vi "MainMesaurementDataPipe.vi"(8 "error in (no error)":errorcluster, 9 "WFChart Refnum":refnum<vi>, 10 "IntGraph Refnum in":refnum<vi>, 11 "IntensityGraph in":refnum<vi>) -> (0 "error out":errorcluster)   [LabVIEW 2013]
uses:
  Variables/GlobalCameraDebugTemperature.vi
  Variables/GlobalGetMesaurementStatus.vi
  Variables/GlobalSetGetPixelOfRoi.vi
  Variables/GlobalDevice.vi
  Variables/GlobalExitVar.vi
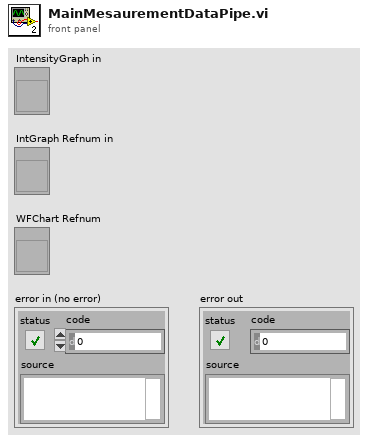
[diagram p1: front panel]
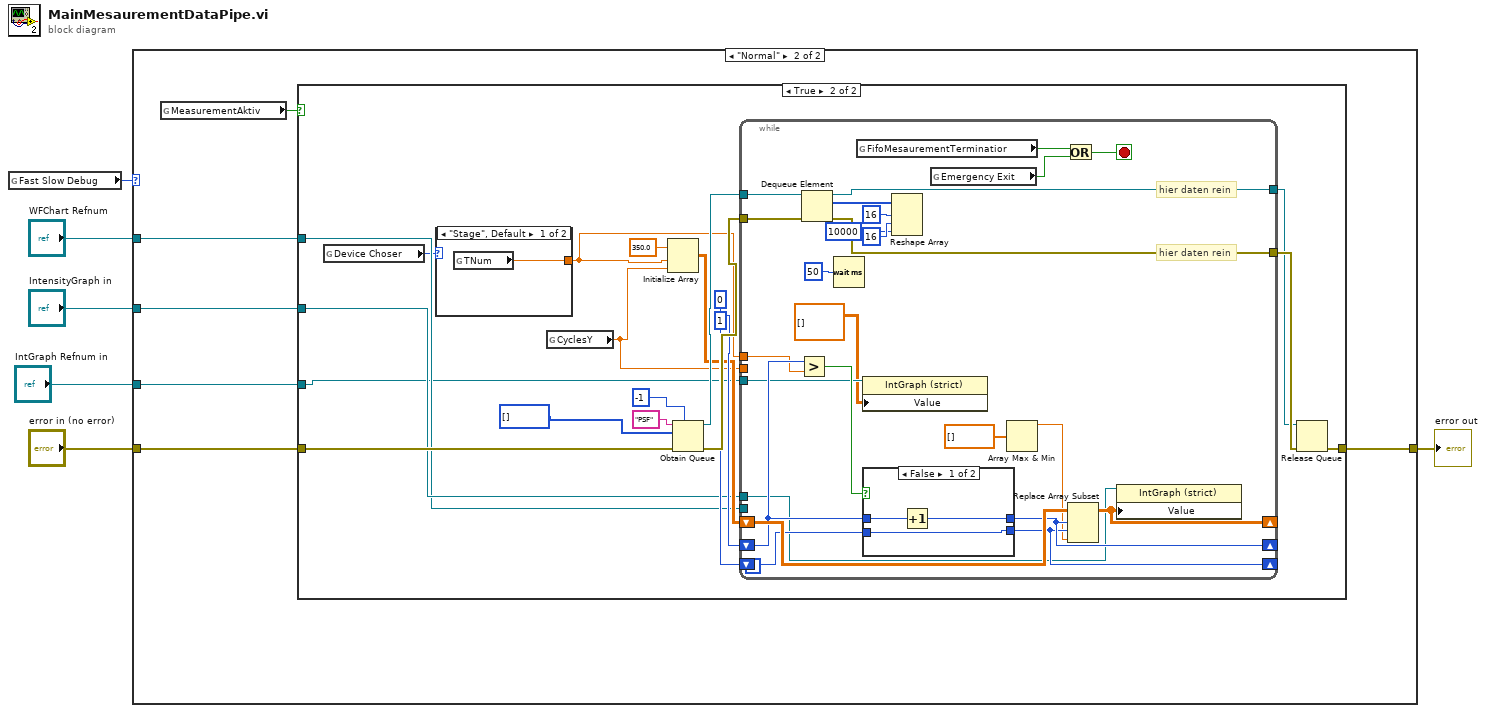
[diagram p0: block diagram]
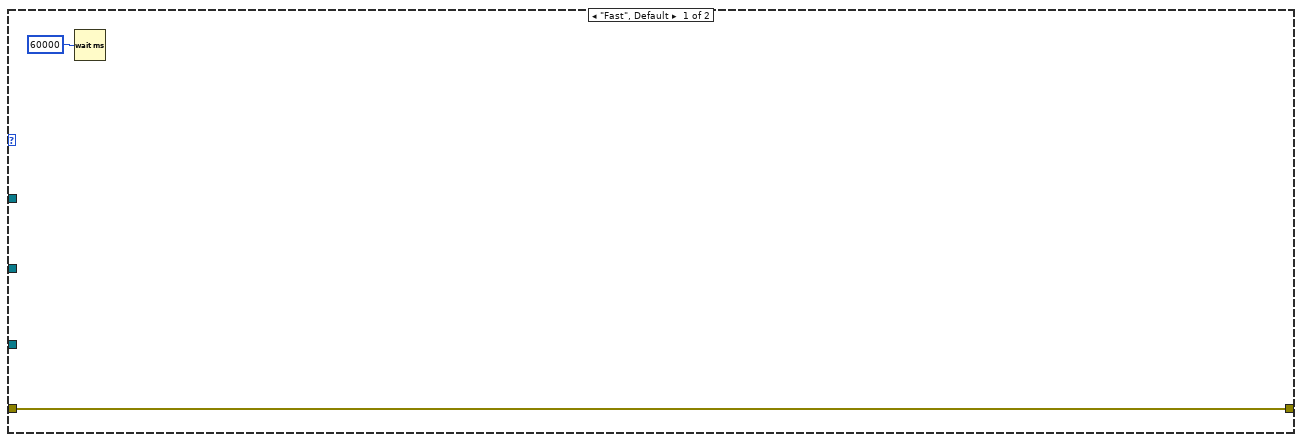
[diagram p2: hidden frame]
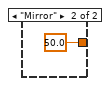
[diagram p4: hidden frame]
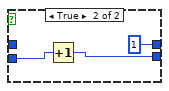
[diagram p5: hidden frame]
diagram:
  n1 = global read "GlobalCameraDebugTemperature.vi" "Fast Slow Debug"() -> (w6:enum32{"Normal", "Fast"})
  n2 = case shown="\"Normal\"" w6 {
    tunnel: [w8 w13] -> w4
    tunnel: "error in (no error)" -> [w8 w12]
    tunnel: "IntensityGraph in" -> [_ w11]
    tunnel: "IntGraph Refnum in" -> [_ w10]
    tunnel: "WFChart Refnum" -> [_ w9]
    frame "Fast", Default {
      n3 = Wait (ms)(milliseconds to wait=u32 60000) -> ()  [unwired: 1 out]
    }
    frame "Normal" {
      n4 = global read "GlobalGetMesaurementStatus.vi" "MeasurementAktiv"() -> (w14:bool)
      n5 = case shown="True" w14 {
        tunnel: [w15 w31] -> w13
        tunnel: w12 -> [w15 w34]
        tunnel: w11 -> [_ w22]
        tunnel: w10 -> [_ w16]
        tunnel: w9 -> [_ w21]
        frame False {
        }
        frame True {
          n6 = global read "GlobalDevice.vi" "Device Choser"() -> (w18:enum32{"Stage", "Mirror"})
          n7 = case shown="\"Stage\", Default" w18 {
            tunnel: [w35 50.0 ("TNum")] -> w20
            frame "Stage", Default {
              n8 = global read "GlobalSetGetPixelOfRoi.vi" "TNum"() -> (w35:dbl)
            }
            frame "Mirror" {
            }
          }
          n9 = global read "GlobalSetGetPixelOfRoi.vi" "CyclesY"() -> (w19:dbl)
          n10 = Initialize Array(350.0 ("element"), w20, w19) -> (w25:dbl[][])
          n11 = Obtain Queue(max queue size (-1, unlimited)=-1, name (unnamed)="PSF", element data type=i32[] [] ("array"), error in (no error)=w34) -> (queue out=w30:refnum<queue>, error out=w33:errorcluster)  [unwired: 1 in, 1 out]
          n12 = while {
            tunnel: w33 -> [w61]
            tunnel: [w60] -> w32
            tunnel: w30 -> [w56]
            tunnel: [w55] -> w29
            shift-right: [w52] -> _
            shift-left: w25 -> [w53]
            tunnel: w20 -> [w49]
            tunnel: w19 -> [_]
            shift-right: [w51] -> _
            shift-left: 0 -> [w50]
            shift-right: [w46] -> _
            shift-left: 1 -> [w47]
            tunnel: w22 -> [w44]
            tunnel: w16 -> [w43]
            tunnel: w21 -> [_]
            stop <- w57 stop-if-true
            # "hier daten rein"
            # "hier daten rein"
            n13 = Greater?(x=w50, y=w49) -> (0:w48:bool)
            n14 = Dequeue Element(queue=w56, error in (no error)=w61) -> (queue out=w55:refnum<queue>, element=w40:i32[], error out=w60:errorcluster)  [unwired: 1 in, 1 out]
            n15 = Wait (ms)(milliseconds to wait=u32 50) -> ()  [unwired: 1 out]
            n16 = global read "GlobalGetMesaurementStatus.vi" "FifoMesaurementTerminatior"() -> (w59:bool)
            n17 = property on="Property Node" class="IntGraph (strict)"(reference=w43, "Value"=dbl[][] []) -> ()  [unwired: 1 in, 2 out]
            n18 = case shown="False" w48 {
              tunnel: [w64 1] -> w51
              tunnel: w50 -> [w63 _]
              tunnel: [w62 w66] -> w46
              tunnel: w47 -> [w62 w65]
              frame False {
                n19 = Increment(x=w63) -> (x+1=w64:i32)
              }
              frame True {
                n20 = Increment(x=w65) -> (x+1=w66:i32)
              }
            }
            n21 = Reshape Array(w40, 16 ("dimension size"), 16 ("dimension size"), 10000 ("dimension size")) -> ()  [unwired: 1 out]
            n22 = global read "GlobalExitVar.vi" "Emergency Exit"() -> (w58:bool)
            n23 = Array Max & Min(array=dbl[] []) -> (max value=w45:dbl)  [unwired: 3 out]
            n24 = Or(x=w59, y=w58) -> (x .or. y?=w57:bool)
            n25 = Replace Array Subset(array=w53, new element=w45, index (row)=w51, index (col)=w46) -> (w52:dbl[][])
            n26 = property on="Property Node" class="IntGraph (strict)"(reference=w44, "Value"=w52) -> ()  [unwired: 1 in, 2 out]
          }
          n27 = Release Queue(queue=w29, error in (no error)=w32) -> (error out=w31:errorcluster)  [unwired: 1 in, 2 out]
        }
      }
    }
  }
  "error out" <- w4
